vi "ChangePWMFrequency.vi"(4 "Frequency (Hz)":dbl=100.0, 5 "Channel":i32, 6 "error in":errorcluster) -> (0 "error out":errorcluster)   [LabVIEW 2014]
doc: "Change the frequency of a channel configured for PWM.\n\nThe channel must be configured for PWM before calling this VI."
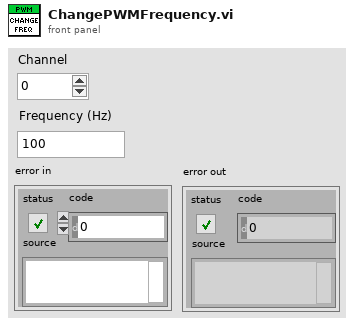
[diagram p1: front panel]
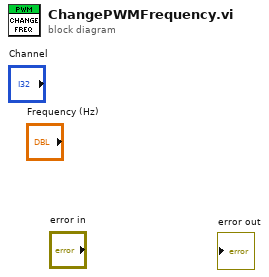
[diagram p0: block diagram]
diagram:
